vi "Read_NIAI.vi"(7 "cnt":T1, 8 "error in":errorcluster) -> (0 "error out":errorcluster, 2 "Array_Data":dbl[](array[numeric]), 3 "data":waveform(dbl)[](graph))   [LabVIEW 2019]
uses:
  cnt_NIAI.ctl
  _ctrl/rw.ctl
  SubVIs/common/cmd_err.ctl
  <vilib>/DAQmx/read.llb/DAQmx Read (Analog 1D Wfm NChan NSamp).vi
  <vilib>/Analysis/baseanly.llb/Mean (DBL).vi
  <vilib>/DAQmx/create/channels.llb/DAQmx Create Channel (AI-Voltage-Basic).vi
  <vilib>/DAQmx/configure/timing.llb/DAQmx Timing (Sample Clock).vi
  <vilib>/DAQmx/miscellaneous.llb/DAQmx Fill In Error Info.vi
  <vilib>/Analysis/NI_AALBase.lvlib
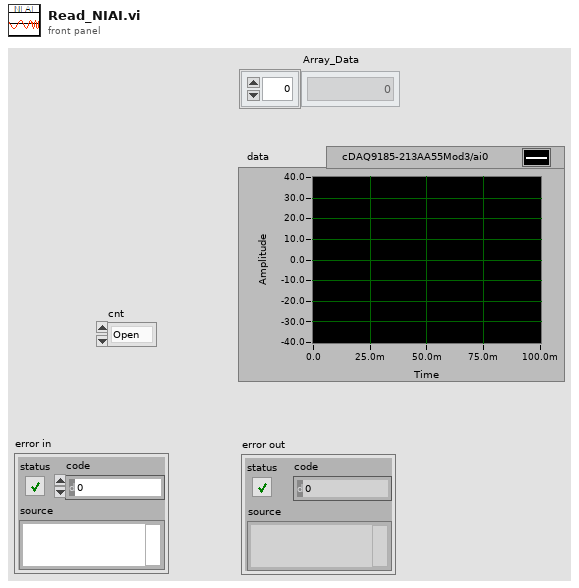
[diagram p1: front panel]
types:
  T1 = typedef "cnt_NIAI.ctl" = enum16{"Open", "Read", "Close"}
  T2 = enum16{"DL950", "BP4610", "DSP1500", "cDAQ-AI", "cDAQ-AO", "cDAQ-DO"}
  T3 = typedef "rw.ctl" = enum16{"read", "write"}
  T4 = typedef "cmd_err.ctl" = enum16{"close", "open", "default"}
  T5 = typedef "Set_NIAI.ctl" = cluster{"input terminal":i32, "minimum value":dbl, "maximum value":dbl, "number of samples":i32, "rate":dbl, "sample mode":i32, "physical channels":tag}
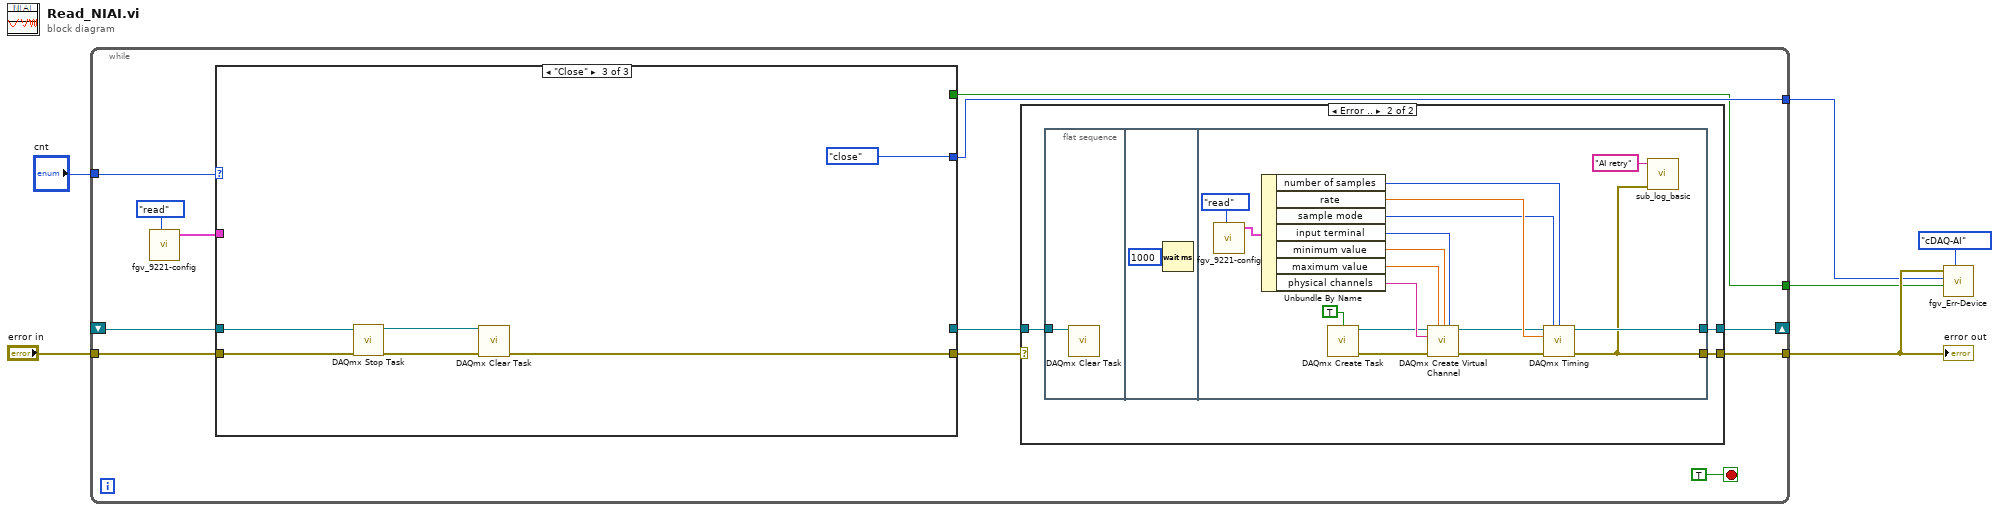
[diagram p0: block diagram]
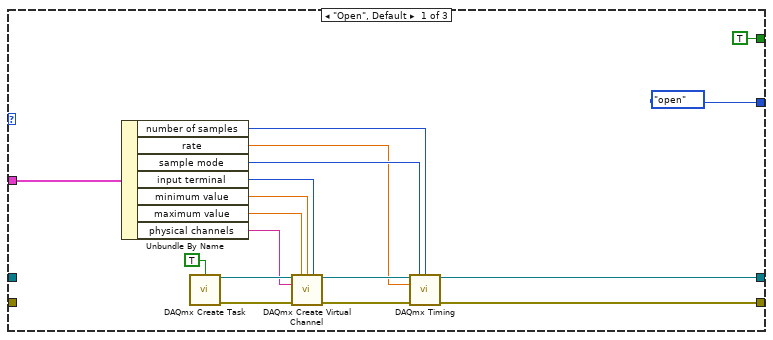
[diagram p3: hidden frame]
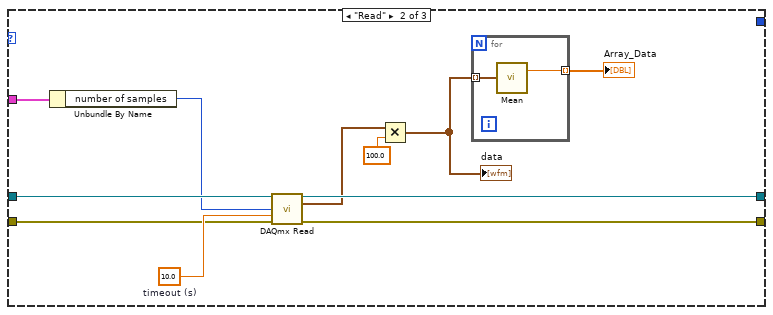
[diagram p4: hidden frame]
diagram:
  n1 = while {
    tunnel: "cnt" -> [w17]
    shift-right: [w10] -> _
    shift-left: _ -> [w16]
    tunnel: "error in" -> [w15]
    tunnel: [w11] -> w3
    tunnel: [w8] -> w2
    tunnel: [w7] -> w1
    stop <- TRUE stop-if-true
    n2 = call "fgv_9221-config.vi"("cmd"=rw."read") -> ("cDAQ 9221 Config 2"=w13:T5)  [unwired: 9 in, 1 out]
    n3 = case shown="\"Close\"" w17 {
      tunnel: [w47 w68 _] -> w9
      tunnel: w16 -> [_ w69 w76]
      tunnel: w15 -> [_ w66 w74]
      tunnel: [w46 w65 w78] -> w12
      tunnel: w13 -> [w45 w64 _]
      tunnel: [cmd_err."open" ("cmd") _ cmd_err."close" ("cmd")] -> w8
      tunnel: [TRUE ("first?") _ _] -> w7
      frame "Open", Default {
        n4 = Unbundle By Name(w45) -> ("number of samples"=w51:i32, "rate"=w49:dbl, "sample mode"=w50:i32, "input terminal"=w55:i32, "minimum value"=w56:dbl, "maximum value"=w57:dbl, "physical channels"=w48:tag)
        n5 = call <vilib>:"DAQmx Create Task.vi"("auto cleanup"=TRUE) -> ("task out"=w58:refnum<k21>, "error out"=w59:errorcluster)  [unwired: 13 in]
        n6 = call-poly <vilib>:"DAQmx Create Virtual Channel.vi"("task in"=w58, "maximum value"=w57, "minimum value"=w56, "input terminal configuration"=w55, "physical channels"=w48, "error in"=w59) -> ("task out"=w53:refnum<k21>, "error out"=w52:errorcluster)  [unwired: 8 in]
        n7 = call-poly <vilib>:"DAQmx Timing.vi"("task/channels in"=w53, "sample mode"=w50, "samples per channel"=w51, "rate"=w49, "error in"=w52) -> ("task out"=w47:refnum<k21>, "error out"=w46:errorcluster)  [unwired: 9 in]
      }
      frame "Read" {
        w70 = 10.0  # timeout (s)
        n8 = Unbundle By Name(w64) -> ("number of samples"=w67:i32)
        n9 = call-poly <vilib>:"DAQmx Read.vi"("task/channels in"=w69, "number of samples per channel"=w67, "timeout"=w70, "error in"=w66) -> ("task out"=w68:refnum<k21>, "data"=w62:waveform(dbl)[], "error out"=w65:errorcluster)  [unwired: 9 in]
        n10 = Multiply(x=w62, y=100.0) -> (x*y=w61:waveform(dbl)[])
        "data" <- w61
        n11 = for {
          tunnel: w61 -> [w72] mode=indexing
          tunnel: [w71] -> w60 mode=indexing
          n12 = call-poly <vilib>:"Mean.vi"("X"=w72) -> ("mean"=w71:dbl)  [unwired: 1 out]
        }
        "Array_Data" <- w60
      }
      frame "Close" {
        n13 = call <vilib>:"DAQmx Stop Task.vi"("task/channels in"=w76, "error in"=w74) -> ("task out"=w75:refnum<k21>, "error out"=w73:errorcluster)  [unwired: 12 in]
        n14 = call <vilib>:"DAQmx Clear Task.vi"("task in"=w75, "error in"=w73) -> ("error out"=w78:errorcluster)  [unwired: 13 in]
      }
    }
    n15 = case shown="Error .." w12 {
      selector: w12 -> [w20 _]
      tunnel: [w20 w21] -> w11
      tunnel: [w19 w22] -> w10
      tunnel: w9 -> [w19 w23]
      frame No Error {
      }
      frame Error {
        n16 = flat-sequence {
          tunnel: w23 -> [w24]
          tunnel: [w28] -> w22
          tunnel: [w26] -> w21
          frame #0 {
            n17 = call <vilib>:"DAQmx Clear Task.vi"("task in"=w24) -> ()  [unwired: 14 in, 1 out]
          }
          frame #1 {
            n18 = Wait (ms)(milliseconds to wait=u32 1000) -> ()  [unwired: 1 out]
          }
          frame #2 {
            n19 = call "fgv_9221-config.vi"("cmd"=rw."read") -> ("cDAQ 9221 Config 2"=w29:T5)  [unwired: 9 in, 1 out]
            n20 = Unbundle By Name(w29) -> ("number of samples"=w39:i32, "rate"=w41:dbl, "sample mode"=w40:i32, "input terminal"=w35:i32, "minimum value"=w34:dbl, "maximum value"=w33:dbl, "physical channels"=w42:tag)
            n21 = call <vilib>:"DAQmx Create Task.vi"("auto cleanup"=TRUE) -> ("task out"=w32:refnum<k21>, "error out"=w31:errorcluster)  [unwired: 13 in]
            n22 = call-poly <vilib>:"DAQmx Create Virtual Channel.vi"("task in"=w32, "maximum value"=w33, "minimum value"=w34, "input terminal configuration"=w35, "physical channels"=w42, "error in"=w31) -> ("task out"=w37:refnum<k21>, "error out"=w38:errorcluster)  [unwired: 8 in]
            n23 = call-poly <vilib>:"DAQmx Timing.vi"("task/channels in"=w37, "sample mode"=w40, "samples per channel"=w39, "rate"=w41, "error in"=w38) -> ("task out"=w28:refnum<k21>, "error out"=w26:errorcluster)  [unwired: 9 in]
            n24 = call "sub_log_basic.vi"("error in"=w26, "Title"="AI retry") -> ()  [unwired: 9 in, 1 out]
          }
        }
      }
    }
  }
  "error out" <- w3
  n25 = call "fgv_Err-Device.vi"("Err Sel"=T2."cDAQ-AI", "first?"=w1, "cmd"=w2, "error in"=w3) -> ()  [unwired: 8 in]
